vi "RSZVB Set Partial Measurement Trigger Mode.vi"(8 "error in (no error)":errorcluster {"code" format="%.0x"}, 9 "Trigger Mode (All Ports)":i32(ring) items=["All Ports", "Port-specific"], 10 "Channel (1)":i32=1, 11 "VISA session":refnum<visa-resource-name>) -> (0 "error out":errorcluster {"code" format="%.0x"}, 3 "dup VISA session":refnum<visa-resource-name>)   [LabVIEW 2011]
doc: "Qualifies whether the trigger delay is valid for all physical ports (including external generator) or source port-specific. This setting is available if the triggered measurement sequence is a partial measurement.\n\nRemote-control command(s):\nTRIGger<Ch>[:SEQuence]:HOLDoff:MODE PALL | PSPecific"
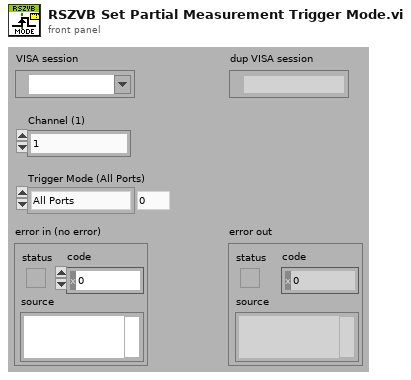
[diagram p1: front panel]
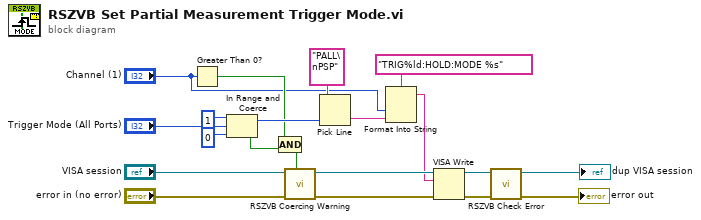
[diagram p0: block diagram]
diagram:
  n1 = Greater Than 0?(x="Channel (1)") -> (x > 0?=w10:bool)
  n2 = In Range and Coerce(upper limit=1, x="Trigger Mode (All Ports)", lower limit=0) -> (coerced(x)=w17:i32, In Range?=w11:bool)
  n3 = Compound Arithmetic op=AND(w10, w11) -> (w9:bool)
  n4 = call "RSZVB Coercing Warning.vi"("In Range?"=w9, "error in (no error)"="error in (no error)", "VISA session"="VISA session") -> ("error out"=w14:errorcluster, "dup VISA session"=w15:refnum<visa-resource-name>)  [unwired: 7 in]
  n5 = Pick Line(multi-line string="PALL\nPSP", line index=w17) -> (output string=w5:string)  [unwired: 1 in]
  n6 = Format Into String(format string="TRIG%ld:HOLD:MODE %s", "Channel (1)", w5) -> (resulting string=w8:string)  [unwired: 2 in, 1 out]
  n7 = VISA Write(VISA resource name=w15, write buffer=w8, error in (no error)=w14) -> (VISA resource name out=w12:refnum<visa-resource-name>, error out=w13:errorcluster)  [unwired: 1 out]
  n8 = call "RSZVB Check Error.vi"("error in (no error)"=w13, "VISA session"=w12) -> ("error out"=→"error out":errorcluster, "dup VISA session"=→"dup VISA session":refnum<visa-resource-name>)  [unwired: 8 in]
